vi "ElliptecRotationAE.vi"(9 "Position or jog size":dbl, 10 "Enum":T1=enum."Read position", 11 "VISA Refnum in":refnum<visa-resource-name>) -> (0 "error out":errorcluster, 1 "String":string, 2 "Read position":i32, 3 "VISA Refnum out":refnum<visa-resource-name>)   [LabVIEW 2022 SP3]
uses:
  D:/Dropbox/Members/Bragg, Alyssa/PolarizerRotator Folder/Control polarizer 1.ctl
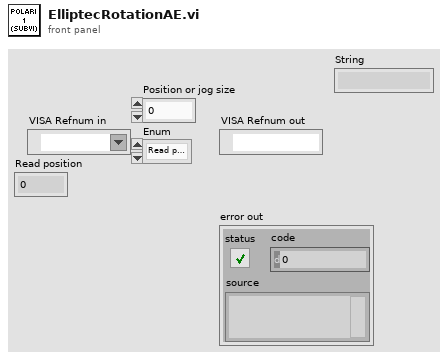
[diagram p1: front panel]
types:
  T1 = typedef "Control polarizer 1.ctl" = enum16{"Home", "Read position", "Go to position", "Jog", "Set jog size"}
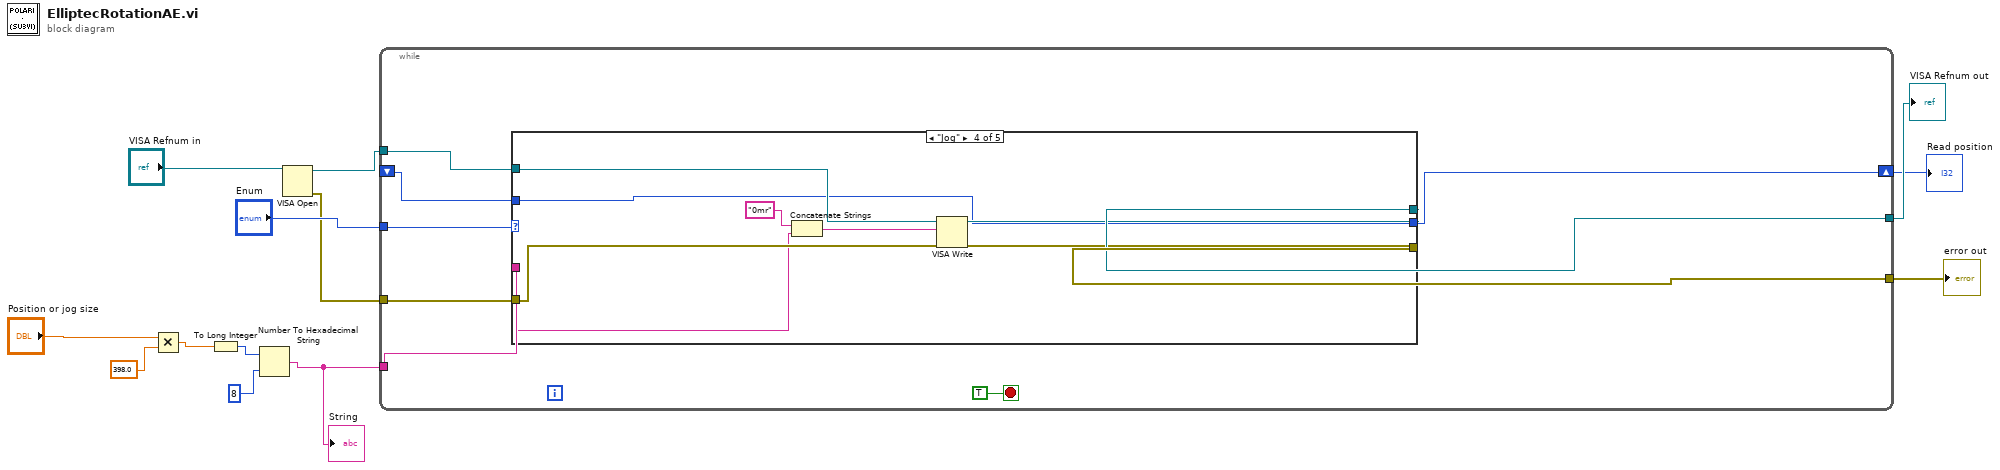
[diagram p0: block diagram]
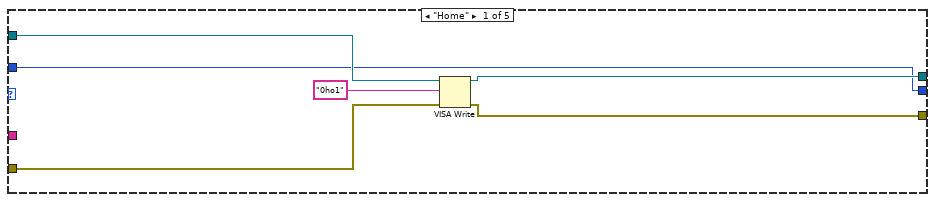
[diagram p2: hidden frame]
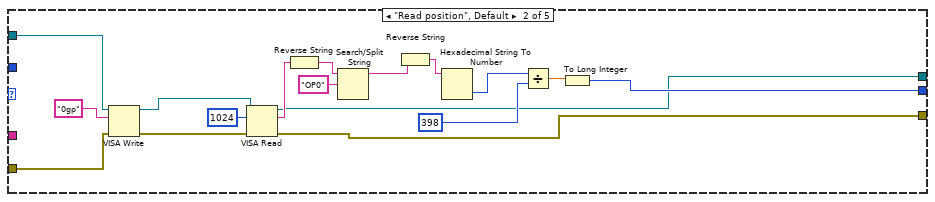
[diagram p3: hidden frame]
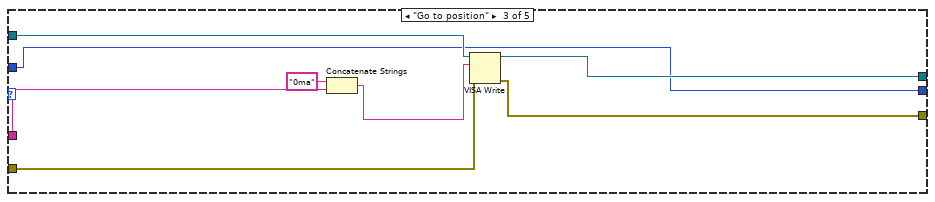
[diagram p4: hidden frame]
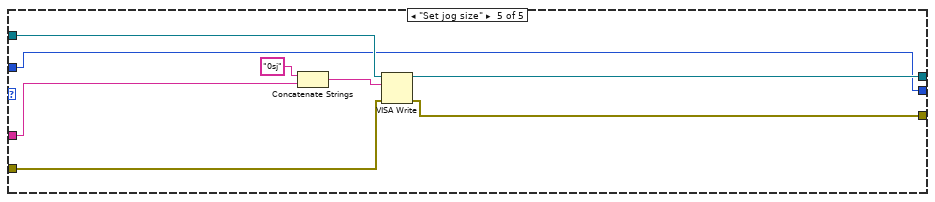
[diagram p5: hidden frame]
diagram:
  n1 = Multiply(x="Position or jog size", y=398.0 ("x")) -> (x*y=w8:dbl)
  n2 = To Long Integer(number=w8) -> (32bit integer=w9:i32)
  n3 = Number To Hexadecimal String(1:i16 8 ("width (-)"), 2:w9) -> (0:w6:string)
  "String" <- w6
  n4 = VISA Open(VISA resource name="VISA Refnum in") -> (VISA resource name=w2:refnum<visa-resource-name>, error out=w1:errorcluster)  [unwired: 4 in]
  n5 = while {
    tunnel: "Enum" -> [w21]
    tunnel: w1 -> [w20]
    tunnel: w2 -> [w19]
    tunnel: [w17] -> w12
    tunnel: [w18] -> w11
    shift-right: [w16] -> w10
    shift-left: _ -> [w15]
    tunnel: w6 -> [w14]
    stop <- TRUE stop-if-true
    n6 = case shown="\"Jog\"" w21 {
      tunnel: w20 -> [w28 w29 w50 w58 w65]
      tunnel: w19 -> [w26 w30 w51 w59 w66]
      tunnel: [w25 w32 w48 w56 w63] -> w18
      tunnel: [w24 w31 w49 w57 w64] -> w17
      tunnel: [w23 w33 w47 w55 w62] -> w16
      tunnel: w15 -> [w23 _ w47 w55 w62]
      tunnel: w14 -> [_ _ w46 w54 w67]
      frame "Home" {
        n7 = VISA Write(VISA resource name=w26, write buffer="0ho1", error in (no error)=w28) -> (VISA resource name out=w24:refnum<visa-resource-name>, error out=w25:errorcluster)  [unwired: 1 out]
      }
      frame "Read position", Default {
        n8 = VISA Write(VISA resource name=w30, write buffer="0gp", error in (no error)=w29) -> (VISA resource name out=w44:refnum<visa-resource-name>, error out=w45:errorcluster)  [unwired: 1 out]
        n9 = VISA Read(VISA resource name=w44, byte count=u32 1024, error in (no error)=w45) -> (VISA resource name out=w31:refnum<visa-resource-name>, read buffer=w43:string, error out=w32:errorcluster)  [unwired: 1 out]
        n10 = Reverse String(1:w43) -> (0:w38:string)
        n11 = Search/Split String(string=w38, search string/char (-)="OP0") -> (substring before match=w39:string)  [unwired: 1 in, 2 out]
        n12 = Reverse String(1:w39) -> (0:w40:string)
        n13 = Hexadecimal String To Number(string=w40) -> (number=w41:u32)  [unwired: 2 in, 1 out]
        n14 = Divide(x=w41, y=u32 398) -> (x/y=w42:dbl)
        n15 = To Long Integer(number=w42) -> (32bit integer=w33:i32)
      }
      frame "Go to position" {
        n16 = Concatenate Strings("0ma" ("string"), w46) -> (w52:string)
        n17 = VISA Write(VISA resource name=w51, write buffer=w52, error in (no error)=w50) -> (VISA resource name out=w49:refnum<visa-resource-name>, error out=w48:errorcluster)  [unwired: 1 out]
      }
      frame "Jog" {
        n18 = Concatenate Strings("0mr" ("write buffer"), w54) -> (w61:string)
        n19 = VISA Write(VISA resource name=w59, write buffer=w61, error in (no error)=w58) -> (VISA resource name out=w57:refnum<visa-resource-name>, error out=w56:errorcluster)  [unwired: 1 out]
      }
      frame "Set jog size" {
        n20 = Concatenate Strings("0sj" ("string"), w67) -> (w68:string)
        n21 = VISA Write(VISA resource name=w66, write buffer=w68, error in (no error)=w65) -> (VISA resource name out=w64:refnum<visa-resource-name>, error out=w63:errorcluster)  [unwired: 1 out]
      }
    }
  }
  "VISA Refnum out" <- w12
  "error out" <- w11
  "Read position" <- w10
